vi "TCP Open Connection PXI.vi"(8 "error in (no error)":errorcluster, 9 "timeout (ms)":i32=5000, 10 "Port":u16=2055 min=1025 step=1, 11 "PXI Address":string="169.254.46.64") -> (0 "error out":errorcluster, 3 "connection ID":refnum<k5>)   [LabVIEW 2015]
uses:
  DAQ Engine VIs/PXI Globals.vi
panel:
  # "Ch3 PXI :169.254.46.64"
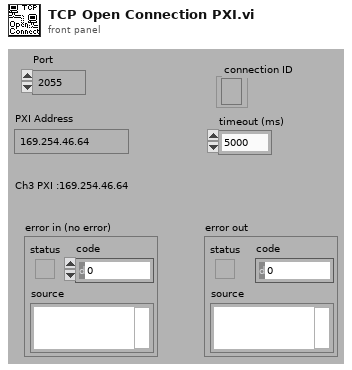
[diagram p1: front panel]
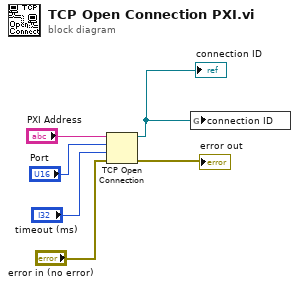
[diagram p0: block diagram]
diagram:
  n1 = TCP Open Connection(address="PXI Address", remote port or service name="Port", timeout ms (60000)="timeout (ms)", error in (no error)="error in (no error)") -> (connection ID=w1:refnum<k5>, error out=→"error out":errorcluster)  [unwired: 1 in]
  "connection ID" <- w1
  n2 = global write "PXI Globals.vi" "connection ID"(w1) -> ()
